vi "To XML - Id is not negative - XML contains id.vi"() -> ()   [LabVIEW 2013, in "JUnit XML Tests.lvlib" / "Test Suite.lvlib"]
uses:
  Test Suite.lvlib
  JUnit XML/Test Suite/Test Suite.lvclass/Test Suite.ctl
  JUnit XML/Test Suite/Test Suite.lvclass
  JUnit XML/Test Suite/Write Timestamp.vi
  <vilib>/xml/Close Reference(Node).vi
  <vilib>/addons/_JKI Toolkits/Caraya/classes/Assert/Assert Equal Value_Variant.vi
  <vilib>/addons/_JKI Toolkits/Caraya/classes/Test/Test.lvclass
  <vilib>/addons/_JKI Toolkits/Caraya/classes/Assert/Assert.lvclass
  <resource>/objmgr/DOMUserDefRef.rc
  <vilib>/xml/NI_XML.lvlib
panel:
  out "error out":errorcluster
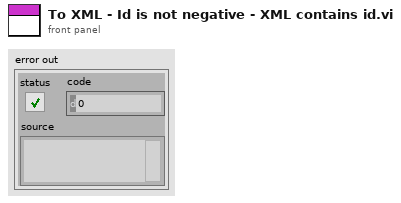
[diagram p1: front panel]
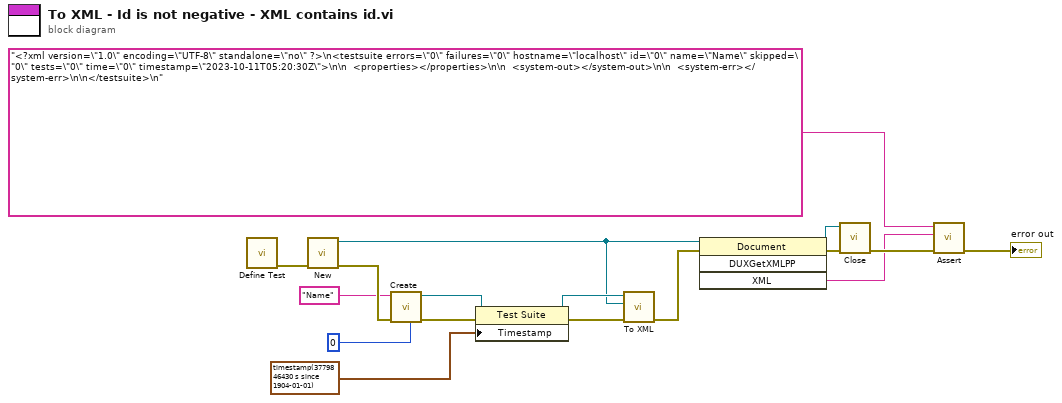
[diagram p0: block diagram]
diagram:
  n1 = call <vilib>:"Define Test.vi"() -> ("error out"=w17:errorcluster)  [unwired: 10 in, 1 out]
  n2 = call <vilib>:"New.vi"("error in (no error)"=w17) -> ("error out"=w15:errorcluster, "DOM document out"=w2:refnum<k20>)  [unwired: 7 in]
  n3 = call "Create.vi"("Id (-1 = undefined)"=0, "error in (no error)"=w15, "Name"="Name" ("Package")) -> ("error out"=w16:errorcluster, "Test Suite"=w7:refnum<class "Test Suite.lvclass">)  [unwired: 7 in]
  n4 = property class="Test Suite"(reference=w7, error in=w16, "Timestamp"=timestamp(3779846430.123 s since 1904-01-01)) -> (reference out=w6:refnum<class "Test Suite.lvclass">, error out=w8:errorcluster)
  n5 = call-dynamic "To XML.vi"("error in (no error)"=w8, "Parent"=w2, "Test Suite in"=w6) -> ("error out"=w1:errorcluster)  [unwired: 8 in]
  n6 = invoke class="Document" method="DUXGetXMLPP"(reference=w2, error in=w1) -> (reference out=w13:refnum<k20>, error out=w14:errorcluster, "XML"=w11:string)  [unwired: 2 in, 1 out]
  n7 = call-poly <vilib>:"Close.vi"("error in (no error)"=w14, "node"=w13) -> ("error out"=w12:errorcluster)  [unwired: 7 in]
  n8 = call-poly <vilib>:"Assert.vi"("error in (no error)"=w12, "Actual"=w11, "Expected"="<?xml version=\"1.0\" encoding=\"UTF-8\" standalone=\"no\" ?>\n<testsuite errors=\"0\" failures=\"0\" hostname=\"localhost\" id=\"0\" name=\"Name\" skipped=\"0\" tests=\"0\" time=\"0\" timestamp=\"2023-10-11T05:20:30Z\">\n\n  <properties></properties>\n\n  <system-out></system-out>\n\n  <system-err></system-err>\n\n</testsuite>\n") -> ("error out"=→"error out":errorcluster)  [unwired: 7 in, 1 out]
